vi "Call WinHelp.vi"(8 "error in (no error)":errorcluster, 10 "search topic":string="Contents", 11 "path to hlp file (lvhelp.hlp)":path) -> (0 "error out":errorcluster)   [LabVIEW 2020, in "MacroAssert.lvlib" / "Winevent.lvlib"]
doc: "Call WinHelp.vi makes a DLL call to the WinHelp function, allowing a search within the any .hlp file for 'search topic'. 'search topic' must be a defined jump-able location within the .hlp file.\n\nIf Path to .hlp file is left empty, the VI finds the labview.hlp file. The VI assumes a standard configuration with the vi.lib and help directories in the same location.\n\nThis VI is presented AS IS.\n\nIf an invalid .hlp file or unknown search topic is entered, the Help engine is started but a dialog box displays a message concerning the problem.\n\nWinHelp supports other search modes. Currently the only mode supported by this VI is to search on a defined search topic. To use other search modes see documentation on WinHelp (MSDN, the MicroSoft Developer's Network, contains information on WinHelp).\n\nROM - 5/95"
uses:
  Winevent.lvlib
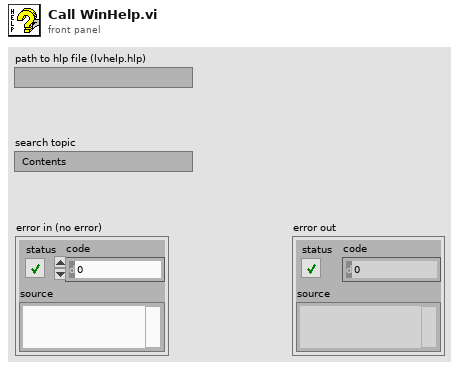
[diagram p1: front panel]
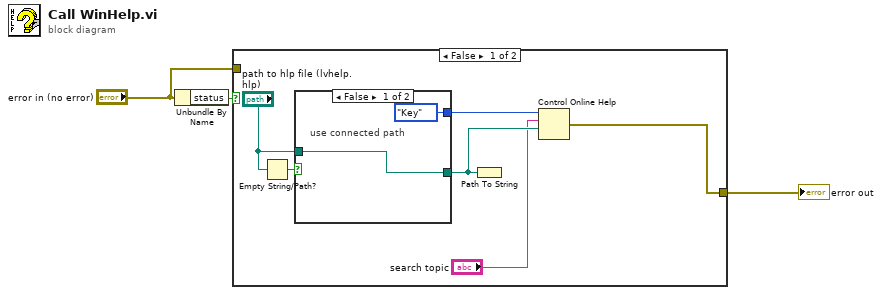
[diagram p0: block diagram]
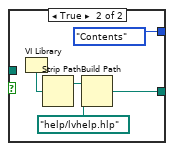
[diagram p2: hidden frame]
diagram:
  n1 = Unbundle By Name("error in (no error)") -> ("status"=w3:bool)
  n2 = case shown="False" w3 {
    tunnel: "error in (no error)" -> [_ w17]
    tunnel: [w4 w17] -> w1
    frame False {
      n3 = Empty String/Path?(string/path="path to hlp file (lvhelp.hlp)") -> (empty?=w8:bool)
      n4 = case shown="False" w8 {
        tunnel: "path to hlp file (lvhelp.hlp)" -> [w11 _]
        tunnel: [w11 w13] -> w7
        tunnel: [enum16{"Contents", "Key", "Close"}."Key" ("Operation") enum16{"Contents", "Key", "Close"}."Contents" ("Operation")] -> w6
        frame False {
          # "use connected path"
        }
        frame True {
          n5 = VI Library() -> (path=w15:path)
          n6 = Strip Path(path=w15) -> (stripped path=w14:path)  [unwired: 1 out]
          n7 = Build Path(base path=w14, name or relative path=path "help/lvhelp.hlp") -> (appended path=w13:path)
        }
      }
      n8 = Path To String(path=w7) -> ()  [unwired: 1 out]
      n9 = Control Online Help(2:w7, 3:"search topic", 4:w6) -> (0:w4:errorcluster)  [unwired: 1 in]
    }
    frame True {
    }
  }
  "error out" <- w1
